vi "Options.vi"(8 "Error In":errorcluster, 11 "Options DVR In":T1) -> (0 "Error Out":errorcluster, 1 "Cancelled?":bool)   [LabVIEW 2011]
uses:
  Controls/Options DVR.ctl
  Controls/Options.ctl
panel:
  in  "Cancel":bool
  in  "OK":bool
  in  "TimeStamp?":bool
  in  "LogDir":path caption="Custom result logging path"
  in  "LogInCSVDir":bool
  in  "Logging":bool
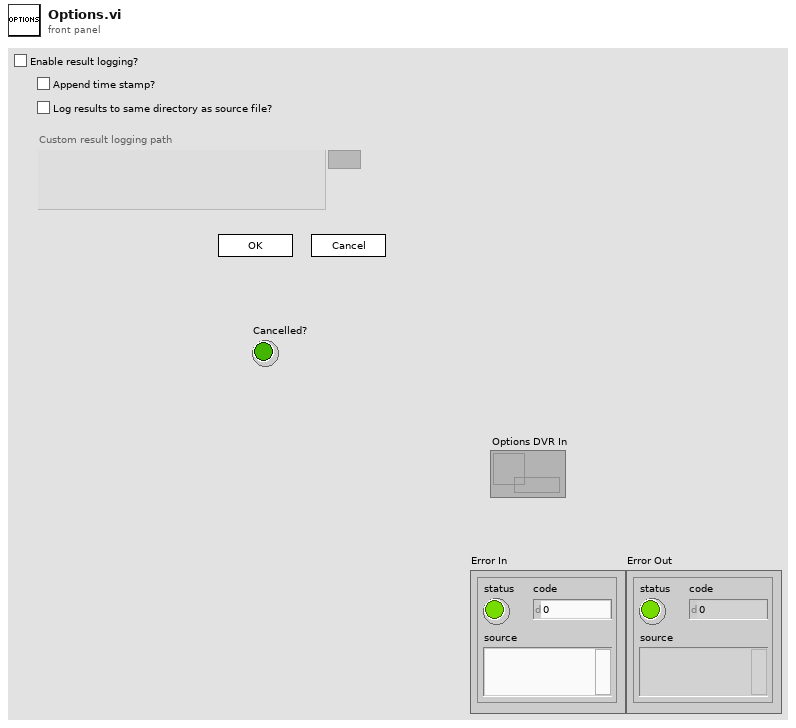
[diagram p1: front panel]
types:
  T1 = typedef "Options DVR.ctl" = refnum<data-value>
  T2 = typedef "Options.ctl" = cluster{"Logging?":bool, "TimeStamp?":bool, "LogInCSVDir?":bool, "LogDir":path}
  T3 = enum8{"Enabled", "Disabled", "Disabled and Grayed Out"}
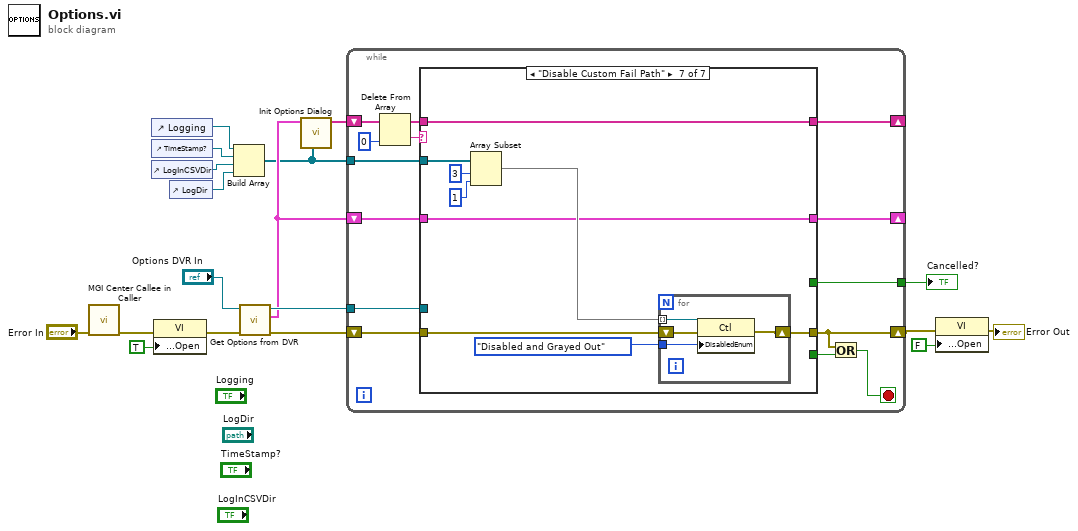
[diagram p0: block diagram]
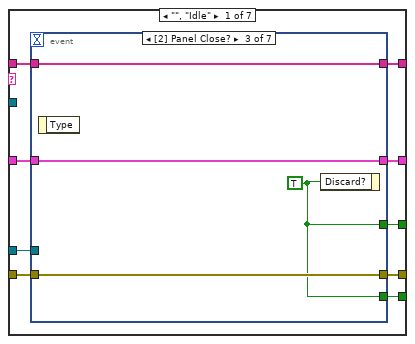
[diagram p2: hidden frame]
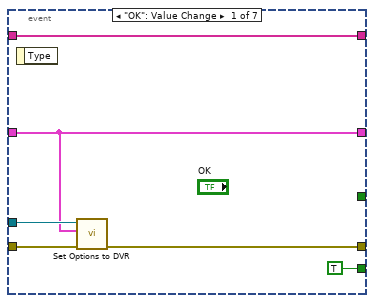
[diagram p3: hidden frame]
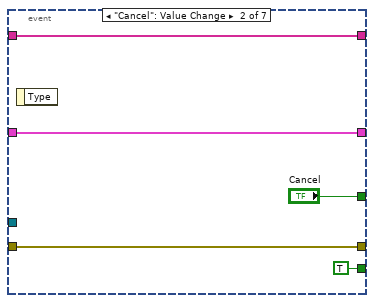
[diagram p4: hidden frame]
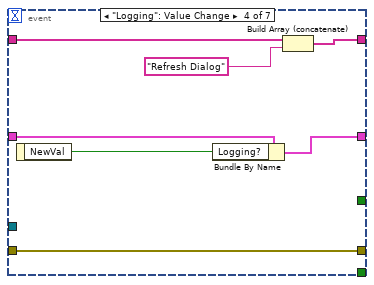
[diagram p5: hidden frame]
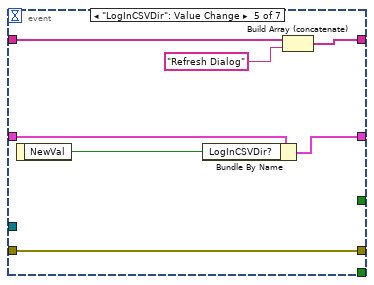
[diagram p6: hidden frame]
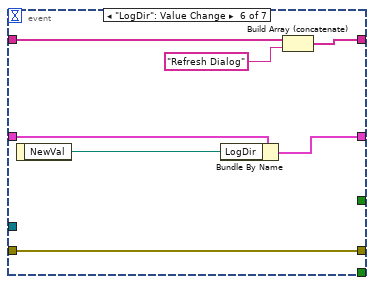
[diagram p7: hidden frame]
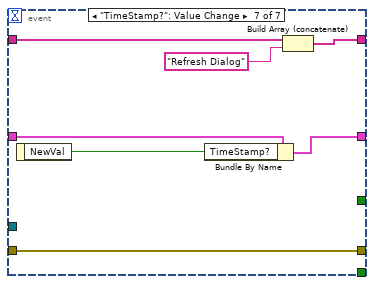
[diagram p8: hidden frame]
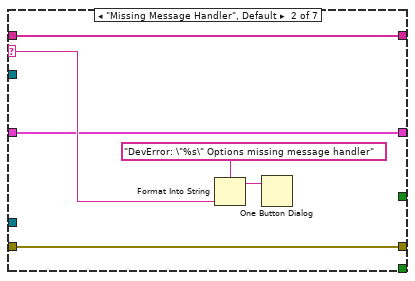
[diagram p9: hidden frame]
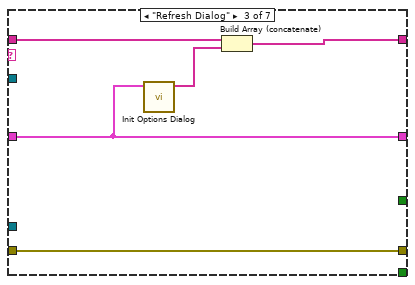
[diagram p10: hidden frame]
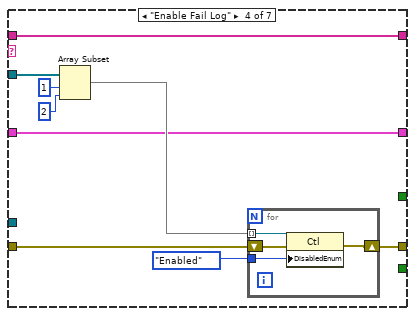
[diagram p11: hidden frame]
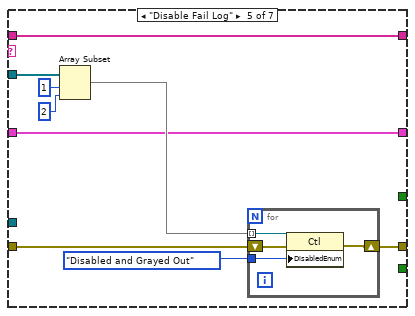
[diagram p12: hidden frame]
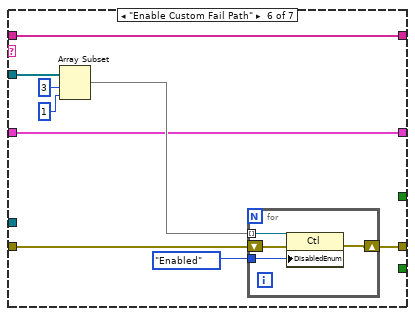
[diagram p13: hidden frame]
diagram:
  n1 = call <userlib>:"MGI Center Callee in Caller.vi"("Error In"="Error In") -> ("Error Out"=w5:errorcluster)  [unwired: 10 in]
  n2 = control-ref of="Logging"() -> (w17:refnum<vi>)
  n3 = control-ref of="TimeStamp?"() -> (w9:refnum<vi>)
  n4 = control-ref of="LogInCSVDir"() -> (w8:refnum<vi>)
  n5 = property on="Property Node" class="VI"(error in=w5, "Front Panel.Open"=TRUE ("Front Panel Window:Open")) -> (error out=w4:errorcluster)  [unwired: 1 in, 1 out]
  n6 = control-ref of="LogDir"() -> (w7:refnum<vi>)
  n7 = Build Array(w17, w9, w8, w7) -> (w12:refnum<vi>[])
  n8 = call "Get Options from DVR.vi"("Error In"=w4, "Options DVR"="Options DVR In") -> ("Error Out"=w16:errorcluster, "Options"=w14:T2, "Options DVR"=w15:T1)  [unwired: 7 in]
  n9 = call "Init Options Dialog.vi"("Controls"=w12, "Options"=w14) -> ("Init Steps"=w13:string[])  [unwired: 9 in]
  n10 = while {
    shift-right: [w22] -> w2
    shift-left: w16 -> [w28]
    shift-right: [w21] -> _
    shift-left: w14 -> [w25]
    shift-right: [w29] -> _
    shift-left: w13 -> [w32]
    tunnel: w12 -> [w27]
    tunnel: w15 -> [w26]
    tunnel: [w19] -> w10
    stop <- w23 stop-if-true
    n11 = Delete From Array(array=w32, index=0) -> (deleted portion=w31:string, array with subset deleted=w30:string[])  [unwired: 1 in]
    n12 = case shown="\"Disable Custom Fail Path\"" w31 {
      selector: w31 -> [_ w87 _ _ _ _ _]
      tunnel: w30 -> [w41 w90 w95 w97 w110 w123 w136]
      tunnel: [w40 w90 w92 w97 w110 w123 w136] -> w29
      tunnel: [w39 w86 w94 w98 w111 w124 w137] -> w22
      tunnel: w28 -> [w38 w86 w94 w101 w114 w127 w140]
      tunnel: w27 -> [_ _ _ w104 w117 w130 w143]
      tunnel: w26 -> [w37 _ _ _ _ _ _]
      tunnel: w25 -> [w36 w85 w93 w96 w109 w122 w135]
      tunnel: [w35 _ _ _ _ _ _] -> w24
      tunnel: [w34 w85 w93 w96 w109 w122 w135] -> w21
      tunnel: [w33 _ _ _ _ _ _] -> w19
      frame "", "Idle" {
        n13 = event shown="[2] Panel Close?" {
          selector: _ -> [_ _ _ _ _ _ _]
          dyn-events: _ -> [_ _ _ _ _ _ _]
          timeout: _ -> [_ _ _ _ _ _ _]
          tunnel: w41 -> [w47 w50 w56 w63 w70 w77 w84]
          tunnel: [w47 w50 w56 w58 w65 w72 w79] -> w40
          tunnel: [w44 w52 w55 w62 w69 w76 w83] -> w39
          tunnel: w38 -> [w46 w52 w55 w62 w69 w76 w83]
          tunnel: w37 -> [w45 _ _ _ _ _ _]
          tunnel: w36 -> [w42 w49 w54 w61 w68 w75 w82]
          tunnel: [TRUE TRUE w53 _ _ _ _] -> w35
          tunnel: [w42 w49 w54 w60 w67 w74 w81] -> w34
          tunnel: [_ "Cancel" w53 _ _ _ _] -> w33
          event "OK": Value Change {
            n14 = event-data() -> ()  [unwired: 1 in, 1 out]
            n15 = call "Set Options to DVR.vi"("Error In"=w46, "Options"=w42, "Options DVR"=w45) -> ("Error Out"=w44:errorcluster)  [unwired: 7 in, 1 out]
          }
          event "Cancel": Value Change {
            n16 = event-data() -> ()  [unwired: 1 in, 1 out]
          }
          event Panel Close? {
            w53 = TRUE ("Discard?")
            n17 = event-data() -> ()  [unwired: 1 in, 1 out]
            n18 = event-data("Discard?"=w53) -> ()  [unwired: 1 in, 1 out]
          }
          event "Logging": Value Change {
            n19 = event-data() -> ("NewVal"=w59:bool)  [unwired: 1 in]
            n20 = Bundle By Name(cluster=w61, "Logging?"=w59) -> (w60:T2)
            n21 = Build Array (concatenate)(w63, "Refresh Dialog") -> (w58:string[])
          }
          event "LogInCSVDir": Value Change {
            n22 = event-data() -> ("NewVal"=w66:bool)  [unwired: 1 in]
            n23 = Bundle By Name(cluster=w68, "LogInCSVDir?"=w66) -> (w67:T2)
            n24 = Build Array (concatenate)(w70, "Refresh Dialog") -> (w65:string[])
          }
          event "LogDir": Value Change {
            n25 = event-data() -> ("NewVal"=w73:path)  [unwired: 1 in]
            n26 = Bundle By Name(cluster=w75, "LogDir"=w73) -> (w74:T2)
            n27 = Build Array (concatenate)(w77, "Refresh Dialog") -> (w72:string[])
          }
          event "TimeStamp?": Value Change {
            n28 = event-data() -> ("NewVal"=w80:bool)  [unwired: 1 in]
            n29 = Bundle By Name(cluster=w82, "TimeStamp?"=w80) -> (w81:T2)
            n30 = Build Array (concatenate)(w84, "Refresh Dialog") -> (w79:string[])
          }
        }
      }
      frame "Missing Message Handler", Default {
        n31 = Format Into String(format string="DevError: \"%s\" Options missing message handler" ("message"), w87) -> (resulting string=w89:string)  [unwired: 2 in, 1 out]
        n32 = One Button Dialog(message=w89) -> ()  [unwired: 2 out]
      }
      frame "Refresh Dialog" {
        n33 = call "Init Options Dialog.vi"("Options"=w93) -> ("Init Steps"=w91:string[])  [unwired: 10 in]
        n34 = Build Array (concatenate)(w95, w91) -> (w92:string[])
      }
      frame "Enable Fail Log" {
        n35 = Array Subset(array=w104, index=1, length=2) -> (w100:refnum<vi>[])
        n36 = for {
          shift-right: [w107] -> w98
          shift-left: w101 -> [w108]
          tunnel: w100 -> [w106] mode=indexing
          tunnel: T3."Enabled" ("Disabled") -> [w105]
          n37 = property class="Ctl"(reference=w106, error in=w108, "DisabledEnum"=w105) -> (error out=w107:errorcluster)  [unwired: 1 out]
        }
      }
      frame "Disable Fail Log" {
        n38 = Array Subset(array=w117, index=1, length=2) -> (w113:refnum<vi>[])
        n39 = for {
          shift-right: [w120] -> w111
          shift-left: w114 -> [w121]
          tunnel: w113 -> [w119] mode=indexing
          tunnel: T3."Disabled and Grayed Out" ("Disabled") -> [w118]
          n40 = property class="Ctl"(reference=w119, error in=w121, "DisabledEnum"=w118) -> (error out=w120:errorcluster)  [unwired: 1 out]
        }
      }
      frame "Enable Custom Fail Path" {
        n41 = Array Subset(array=w130, index=3, length=1) -> (w126:refnum<vi>[])
        n42 = for {
          shift-right: [w133] -> w124
          shift-left: w127 -> [w134]
          tunnel: w126 -> [w132] mode=indexing
          tunnel: T3."Enabled" ("Disabled") -> [w131]
          n43 = property class="Ctl"(reference=w132, error in=w134, "DisabledEnum"=w131) -> (error out=w133:errorcluster)  [unwired: 1 out]
        }
      }
      frame "Disable Custom Fail Path" {
        n44 = Array Subset(array=w143, index=3, length=1) -> (w139:refnum<vi>[])
        n45 = for {
          shift-right: [w146] -> w137
          shift-left: w140 -> [w147]
          tunnel: w139 -> [w145] mode=indexing
          tunnel: T3."Disabled and Grayed Out" ("Disabled") -> [w144]
          n46 = property class="Ctl"(reference=w145, error in=w147, "DisabledEnum"=w144) -> (error out=w146:errorcluster)  [unwired: 1 out]
        }
      }
    }
    n47 = Or(x=w22, y=w24) -> (x .or. y?=w23:bool)
  }
  "Cancelled?" <- w10
  n48 = property on="Property Node" class="VI"(error in=w2, "Front Panel.Open"=FALSE ("Front Panel Window:Open")) -> (error out=→"Error Out":errorcluster)  [unwired: 1 in, 1 out]
